vi "メイン.vi"() -> (2 "測定周期/ms":dbl, 3 "値転記用配列":T2[](array[typedef]))   [LabVIEW 2021] (continued)
                          n2295 = Add(x=w4469, y=13) -> (x+y=w4460:i32)
                          n2296 = local read "csv作成表"() -> (w4456:string[][])
                          n2297 = Unbundle By Name(w4467) -> ("実測値(MAX)"=w4463:string, "実測値(MIN)"=w4464:string)
                          n2298 = Replace Array Subset(array=w4456, new element #1=w4463, index (row) #1=w4461, index (col) #1=w4462, new element #2=w4464, index (row) #2=w4461, index (col) #2=w4460) -> (w4458:string[][])
                          n2299 = Select(t=w4458, s=w4468, f=w4456) -> (s? t:f=w4459:string[][])
                          n2300 = local write "csv作成表"(w4459) -> ()
                        }
                        frame 11 {
                          w4479 = 2
                          # "B"
                          # "A"
                          # "csv作成の為表へクラスタ(実測値)書き込み"
                          # "⑤"
                          # "③"
                          # "④"
                          n2301 = local read "メインON/OFF_\n設定 12"() -> (w4490:T1)
                          n2302 = Unbundle By Name(w4490) -> ("使用ON/OFF"=w4486:bool)
                          n2303 = control-ref of="前回値転記用配列"() -> (w4484:refnum<vi>)
                          n2304 = local read "メイン設定_設定 12"() -> (w4491:T2)
                          n2305 = call "メイン_測定値配列_CSV転記サブ.vi"("メイン設定_設定入力"=w4491, "ループ反復数値入力"=w4488, "実測設定項目"=w4489, "使用ON/OFF"=w4486, "前回値転記用配列"=w4484) -> ("ループ反復数値出力"=w4487:i32, "メイン設定_設定出力"=w4485:T2)  [unwired: 5 in]
                          n2306 = local write "メイン設定_設定 12"(w4485) -> ()
                          n2307 = Add(x=13, y=w4487) -> (x+y=w4480:i32)
                          n2308 = Add(x=w4487, y=14) -> (x+y=w4478:i32)
                          n2309 = local read "csv作成表"() -> (w4474:string[][])
                          n2310 = Unbundle By Name(w4485) -> ("実測値(MAX)"=w4481:string, "実測値(MIN)"=w4482:string)
                          n2311 = Replace Array Subset(array=w4474, new element #1=w4481, index (row) #1=w4479, index (col) #1=w4480, new element #2=w4482, index (row) #2=w4479, index (col) #2=w4478) -> (w4476:string[][])
                          n2312 = Select(t=w4476, s=w4486, f=w4474) -> (s? t:f=w4477:string[][])
                          n2313 = local write "csv作成表"(w4477) -> ()
                        }
                      }
                    }
                  }
                }
                n2314 = local write "値転記用配列"(w4248) -> ()
                n2315 = flat-sequence {
                  tunnel: [w4263] -> w4249
                  tunnel: w4248 -> [w4263]
                  frame #0 {
                    w4258 = T9 {"Horizontal"=-51, "Vertical"=216} ("座標 3")
                    n2316 = control-ref of="このVI"() -> (w4259:refnum<vi>)
                    n2317 = property on="ペーン 2" class="Pane"("Origin"=w4258) -> ()  [unwired: 2 in, 2 out]
                    n2318 = property on="ペーン 2" class="Pane"("Origin"=w4258) -> ()  [unwired: 2 in, 2 out]
                    n2319 = control-ref of="このVI"() -> (w4261:refnum<vi>)
                    n2320 = Unbundle(w4258) -> ("Vertical"=w4260:i16)  [unwired: 1 out]
                    n2321 = Unbundle(w4258) -> ("Vertical"=w4262:i16)  [unwired: 1 out]
                    n2322 = call "メイン_装飾移動サブ.vi"("Y軸座標入力"=w4260, "VI入力"=w4259) -> ()  [unwired: 10 in]
                    n2323 = call "メイン_装飾枠移動サブ.vi"("Y軸座標入力"=w4262, "VI入力"=w4261) -> ()  [unwired: 10 in]
                  }
                }
              }
              frame #1 {
                w4493 = T8."Enabled" ("無効")
                # "⑪ボタンの無効解除"
                n2324 = for {
                  N: 12 -> [_]
                  tunnel: w4493 -> [w4496]
                  i -> [w4497]
                  n2325 = case shown="11" w4497 {
                    tunnel: w4496 -> [w4498 w4499 w4500 w4501 w4502 w4503 w4504 w4505 w4506 w4507 w4508 w4509]
                    frame 0, Default {
                      n2326 = property on="メイン測定ボタン_単発 1" class="Bool (指定)"("DisabledEnum"=w4498) -> ()  [unwired: 2 in, 2 out]
                      n2327 = property on="メイン測定ボタン_連続 1" class="Bool (指定)"("DisabledEnum"=w4498) -> ()  [unwired: 2 in, 2 out]
                    }
                    frame 1 {
                      n2328 = property on="メイン測定ボタン_単発 2" class="Bool (指定)"("DisabledEnum"=w4499) -> ()  [unwired: 2 in, 2 out]
                      n2329 = property on="メイン測定ボタン_連続 2" class="Bool (指定)"("DisabledEnum"=w4499) -> ()  [unwired: 2 in, 2 out]
                    }
                    frame 2 {
                      n2330 = property on="メイン測定ボタン_単発 3" class="Bool (指定)"("DisabledEnum"=w4500) -> ()  [unwired: 2 in, 2 out]
                      n2331 = property on="メイン測定ボタン_連続 3" class="Bool (指定)"("DisabledEnum"=w4500) -> ()  [unwired: 2 in, 2 out]
                    }
                    frame 3 {
                      n2332 = property on="メイン測定ボタン_単発 4" class="Bool (指定)"("DisabledEnum"=w4501) -> ()  [unwired: 2 in, 2 out]
                      n2333 = property on="メイン測定ボタン_連続 4" class="Bool (指定)"("DisabledEnum"=w4501) -> ()  [unwired: 2 in, 2 out]
                    }
                    frame 4 {
                      n2334 = property on="メイン測定ボタン_単発 5" class="Bool (指定)"("DisabledEnum"=w4502) -> ()  [unwired: 2 in, 2 out]
                      n2335 = property on="メイン測定ボタン_連続 5" class="Bool (指定)"("DisabledEnum"=w4502) -> ()  [unwired: 2 in, 2 out]
                    }
                    frame 5 {
                      n2336 = property on="メイン測定ボタン_連続 6" class="Bool (指定)"("DisabledEnum"=w4503) -> ()  [unwired: 2 in, 2 out]
                      n2337 = property on="メイン測定ボタン_単発 6" class="Bool (指定)"("DisabledEnum"=w4503) -> ()  [unwired: 2 in, 2 out]
                    }
                    frame 6 {
                      n2338 = property on="メイン測定ボタン_連続 7" class="Bool (指定)"("DisabledEnum"=w4504) -> ()  [unwired: 2 in, 2 out]
                      n2339 = property on="メイン測定ボタン_単発 7" class="Bool (指定)"("DisabledEnum"=w4504) -> ()  [unwired: 2 in, 2 out]
                    }
                    frame 7 {
                      n2340 = property on="メイン測定ボタン_単発 8" class="Bool (指定)"("DisabledEnum"=w4505) -> ()  [unwired: 2 in, 2 out]
                      n2341 = property on="メイン測定ボタン_連続 8" class="Bool (指定)"("DisabledEnum"=w4505) -> ()  [unwired: 2 in, 2 out]
                    }
                    frame 8 {
                      n2342 = property on="メイン測定ボタン_単発 9" class="Bool (指定)"("DisabledEnum"=w4506) -> ()  [unwired: 2 in, 2 out]
                      n2343 = property on="メイン測定ボタン_連続 9" class="Bool (指定)"("DisabledEnum"=w4506) -> ()  [unwired: 2 in, 2 out]
                    }
                    frame 9 {
                      n2344 = property on="メイン測定ボタン_単発 10" class="Bool (指定)"("DisabledEnum"=w4507) -> ()  [unwired: 2 in, 2 out]
                      n2345 = property on="メイン測定ボタン_連続 10" class="Bool (指定)"("DisabledEnum"=w4507) -> ()  [unwired: 2 in, 2 out]
                    }
                    frame 10 {
                      n2346 = property on="メイン測定ボタン_単発 11" class="Bool (指定)"("DisabledEnum"=w4508) -> ()  [unwired: 2 in, 2 out]
                      n2347 = property on="メイン測定ボタン_連続 11" class="Bool (指定)"("DisabledEnum"=w4508) -> ()  [unwired: 2 in, 2 out]
                    }
                    frame 11 {
                      n2348 = property on="メイン測定ボタン_連続 12" class="Bool (指定)"("DisabledEnum"=w4509) -> ()  [unwired: 2 in, 2 out]
                      n2349 = property on="メイン測定ボタン_単発 12" class="Bool (指定)"("DisabledEnum"=w4509) -> ()  [unwired: 2 in, 2 out]
                    }
                  }
                }
                n2350 = local write "測定新値\nリセット用 4"(TRUE) -> ()
                n2351 = property on="TOPページへ" class="Bool"("DisabledEnum"=w4493) -> ()  [unwired: 2 in, 2 out]
                n2352 = property on="保存して終了" class="Bool"("DisabledEnum"=w4493) -> ()  [unwired: 2 in, 2 out]
                n2353 = property on="保存せずに" class="Bool"("DisabledEnum"=w4493) -> ()  [unwired: 2 in, 2 out]
              }
            }
          }
          frame True {
          }
        }
      }
      frame "測定5" {
        # "⑦"
        # "項目別のボタンで測定を行う為、項目分必要"
        n2354 = local read "測定旧値 5"() -> (w4513:bool)
        n2355 = case shown="FALSE" w4513 {
          tunnel: w4511 -> [w4516 w4779]
          tunnel: [w4515 w4779] -> w4512
          frame False {
            n2356 = flat-sequence {
              tunnel: w4516 -> [w4526]
              tunnel: [w4518] -> w4514
              tunnel: [w4764] -> w4515
              tunnel: w4514 -> [w4764]
              frame #0 {
                # "※複製コピー時変更する項目\n①②\nローカル変数\n\n入れ子のケースストラクチャ\"2\"を複製\n\n0～数だけ変更する\n③④⑤\nローカル変数\n\n※AB\n行番号の変更をする必要がある\n\n--------------------------------\nこの後イベントストラクチャ複製する\n--------------------------------\nイベントストラクチャ複製後\n\n⑦⑧\nローカル変数\n⑨\n装飾体の位置設定\n-51は固定\n前ケースの数値+72\n⑩\n測定新値リセット用\nのボタンが複製されているので、\nフロントパネルを整理する\n⑪\nプロパティノード\nボタンの無効解除クリア以外全てのボタン対象"
                # "実測完了の簡易疑似コード\n\n1)測定モードが単発・連続、多点かで転記する配列を変える\n2)値転記用配列へ転記\n\nここからゲージ分を繰り返す必要がある\n\n3)配列0を取り出す\n4)配列0のポートNoを取り出す\n5)メイン測定_設定配列(測定1の対象配列)のポートNoと比較\n6)同じだったら処理をする。違ったら何もしない\n7)同じだったら配列0のメインON/OFF_設定1の使用ON/OFFがTrueかFalseか\nFlaseだったら前回値転記用配列から前回の値をメイン設定_設定へ転記\nTrueだったらメイン設定_設定の測定モードから\n0単発、1連続、3多点\nの処理を行う\n8)測定値をメイン設定_設定へ転記したら、前回転記用配列へ転記する"
                # "⑨"
                # "⑧"
                # "②"
                # "グループNO(表示上はポートNo)が同じだったら値を転記する\n\n測定した配列のグループNOと値転記用配列の他の指標グループNOを比較する\n＝だったら、対象の配列のON/OFFボタンがTrueか確認し、\nTrueだったら、測定モードによって、値かMAX、MINの数値を転記する\n\nグループNOが同じでなければ、転記しない(何もしない)"
                # "まず値転記用配列に測定の値を転記"
                # "実測定画面vi動作"
                n2357 = local read "メイン設定_設定 5"() -> (w4521:T2)
                n2358 = local read "測定新値 5"() -> (→"測定新値\nリセット用 5":bool)
                n2359 = local read "測定周期/ms"() -> (w4519:dbl)
                n2360 = Unbundle By Name(w4521) -> ("測定モード"=w4522:u16)
                n2361 = call "実測定画面.vi"("実測設定項目配列_\nメインからの転記"=w4526, "測定周期/ms_制御器"=w4519) -> ("実測設定項目配列_\nゲージIOへ転記用"=w4524:T2[], "実測設定項目配列_\n多点測定メイン転記用"=w4523:T2[])  [unwired: 11 in, 1 out]
                n2362 = case shown="1" w4522 {
                  tunnel: w4524 -> [w4533 w4534 _]
                  tunnel: [w4533 w4534 w4535] -> w4517
                  tunnel: w4523 -> [_ _ w4535]
                  frame 0, Default {
                  }
                  frame 1 {
                  }
                  frame 2 {
                  }
                }
                n2363 = for {
                  N: 32 -> [_]
                  tunnel: w4517 -> [w4542]
                  i -> [w4537]
                  # "①"
                  # "※複製コピーはこのケースで行う"
                  # "32回分"
                  # "比較する固定GNO"
                  n2364 = local read "メイン設定_設定 5"() -> (w4536:T2)
                  n2365 = Index Array(array=w4542, index=w4537) -> (element=w4541:T2)
                  n2366 = Unbundle By Name(w4536) -> ("ポートNo."=w4540:dbl)
                  n2367 = Unbundle By Name(w4541) -> ("ポートNo."=w4539:dbl)
                  n2368 = Equal?(x=w4540, y=w4539) -> (x = y?=w4538:bool)
                  n2369 = case shown="TRUE" w4538 {
                    tunnel: w4541 -> [_ w4544]
                    tunnel: w4537 -> [_ w4543]
                    frame False {
                    }
                    frame True {
                      n2370 = case shown="0, デフォルト" w4543 {
                        tunnel: w4544 -> [w4560 w4578 w4596 w4614 w4632 w4650 w4668 w4686 w4704 w4722 w4740 w4758]
                        tunnel: w4543 -> [w4559 w4577 w4595 w4613 w4631 w4649 w4667 w4685 w4703 w4721 w4739 w4757]
                        frame 0, Default {
                          w4550 = 2
                          # "B"
                          # "A"
                          # "csv作成の為表へクラスタ(実測値)書き込み"
                          # "⑤"
                          # "③"
                          # "④"
                          n2371 = local read "メインON/OFF_\n設定 1"() -> (w4561:T1)
                          n2372 = Unbundle By Name(w4561) -> ("使用ON/OFF"=w4557:bool)
                          n2373 = control-ref of="前回値転記用配列"() -> (w4555:refnum<vi>)
                          n2374 = local read "メイン設定_設定 1"() -> (w4562:T2)
                          n2375 = call "メイン_測定値配列_CSV転記サブ.vi"("メイン設定_設定入力"=w4562, "ループ反復数値入力"=w4559, "実測設定項目"=w4560, "使用ON/OFF"=w4557, "前回値転記用配列"=w4555) -> ("ループ反復数値出力"=w4558:i32, "メイン設定_設定出力"=w4556:T2)  [unwired: 5 in]
                          n2376 = local write "メイン設定_設定 1"(w4556) -> ()
                          n2377 = Add(x=2, y=w4558) -> (x+y=w4551:i32)
                          n2378 = Add(x=w4558, y=3) -> (x+y=w4549:i32)
                          n2379 = local read "csv作成表"() -> (w4545:string[][])
                          n2380 = Unbundle By Name(w4556) -> ("実測値(MAX)"=w4552:string, "実測値(MIN)"=w4553:string)
                          n2381 = Replace Array Subset(array=w4545, new element #1=w4552, index (row) #1=w4550, index (col) #1=w4551, new element #2=w4553, index (row) #2=w4550, index (col) #2=w4549) -> (w4547:string[][])
                          n2382 = Select(t=w4547, s=w4557, f=w4545) -> (s? t:f=w4548:string[][])
                          n2383 = local write "csv作成表"(w4548) -> ()
                        }
                        frame 1 {
                          w4568 = 2
                          # "B"
                          # "A"
                          # "csv作成の為表へクラスタ(実測値)書き込み"
                          # "⑤"
                          # "③"
                          # "④"
                          n2384 = local read "メインON/OFF_\n設定 2"() -> (w4579:T1)
                          n2385 = Unbundle By Name(w4579) -> ("使用ON/OFF"=w4575:bool)
                          n2386 = control-ref of="前回値転記用配列"() -> (w4573:refnum<vi>)
                          n2387 = local read "メイン設定_設定 2"() -> (w4580:T2)
                          n2388 = call "メイン_測定値配列_CSV転記サブ.vi"("メイン設定_設定入力"=w4580, "ループ反復数値入力"=w4577, "実測設定項目"=w4578, "使用ON/OFF"=w4575, "前回値転記用配列"=w4573) -> ("ループ反復数値出力"=w4576:i32, "メイン設定_設定出力"=w4574:T2)  [unwired: 5 in]
                          n2389 = local write "メイン設定_設定 2"(w4574) -> ()
                          n2390 = Add(x=3, y=w4576) -> (x+y=w4569:i32)
                          n2391 = Add(x=w4576, y=4) -> (x+y=w4567:i32)
                          n2392 = local read "csv作成表"() -> (w4563:string[][])
                          n2393 = Unbundle By Name(w4574) -> ("実測値(MAX)"=w4570:string, "実測値(MIN)"=w4571:string)
                          n2394 = Replace Array Subset(array=w4563, new element #1=w4570, index (row) #1=w4568, index (col) #1=w4569, new element #2=w4571, index (row) #2=w4568, index (col) #2=w4567) -> (w4565:string[][])
                          n2395 = Select(t=w4565, s=w4575, f=w4563) -> (s? t:f=w4566:string[][])
                          n2396 = local write "csv作成表"(w4566) -> ()
                        }
                        frame 2 {
                          w4586 = 2
                          # "B"
                          # "A"
                          # "csv作成の為表へクラスタ(実測値)書き込み"
                          # "⑤"
                          # "③"
                          # "④"
                          n2397 = local read "メインON/OFF_\n設定 3"() -> (w4597:T1)
                          n2398 = Unbundle By Name(w4597) -> ("使用ON/OFF"=w4593:bool)
                          n2399 = control-ref of="前回値転記用配列"() -> (w4591:refnum<vi>)
                          n2400 = local read "メイン設定_設定 3"() -> (w4598:T2)
                          n2401 = call "メイン_測定値配列_CSV転記サブ.vi"("メイン設定_設定入力"=w4598, "ループ反復数値入力"=w4595, "実測設定項目"=w4596, "使用ON/OFF"=w4593, "前回値転記用配列"=w4591) -> ("ループ反復数値出力"=w4594:i32, "メイン設定_設定出力"=w4592:T2)  [unwired: 5 in]
                          n2402 = local write "メイン設定_設定 3"(w4592) -> ()
                          n2403 = Add(x=4, y=w4594) -> (x+y=w4587:i32)
                          n2404 = Add(x=w4594, y=5) -> (x+y=w4585:i32)
                          n2405 = local read "csv作成表"() -> (w4581:string[][])
                          n2406 = Unbundle By Name(w4592) -> ("実測値(MAX)"=w4588:string, "実測値(MIN)"=w4589:string)
                          n2407 = Replace Array Subset(array=w4581, new element #1=w4588, index (row) #1=w4586, index (col) #1=w4587, new element #2=w4589, index (row) #2=w4586, index (col) #2=w4585) -> (w4583:string[][])
                          n2408 = Select(t=w4583, s=w4593, f=w4581) -> (s? t:f=w4584:string[][])
                          n2409 = local write "csv作成表"(w4584) -> ()
                        }
                        frame 3 {
                          w4604 = 2
                          # "B"
                          # "A"
                          # "csv作成の為表へクラスタ(実測値)書き込み"
                          # "⑤"
                          # "③"
                          # "④"
                          n2410 = local read "メインON/OFF_\n設定 4"() -> (w4615:T1)
                          n2411 = Unbundle By Name(w4615) -> ("使用ON/OFF"=w4611:bool)
                          n2412 = control-ref of="前回値転記用配列"() -> (w4609:refnum<vi>)
                          n2413 = local read "メイン設定_設定 4"() -> (w4616:T2)
                          n2414 = call "メイン_測定値配列_CSV転記サブ.vi"("メイン設定_設定入力"=w4616, "ループ反復数値入力"=w4613, "実測設定項目"=w4614, "使用ON/OFF"=w4611, "前回値転記用配列"=w4609) -> ("ループ反復数値出力"=w4612:i32, "メイン設定_設定出力"=w4610:T2)  [unwired: 5 in]
                          n2415 = local write "メイン設定_設定 4"(w4610) -> ()
                          n2416 = Add(x=5, y=w4612) -> (x+y=w4605:i32)
                          n2417 = Add(x=w4612, y=6) -> (x+y=w4603:i32)
                          n2418 = local read "csv作成表"() -> (w4599:string[][])
                          n2419 = Unbundle By Name(w4610) -> ("実測値(MAX)"=w4606:string, "実測値(MIN)"=w4607:string)
                          n2420 = Replace Array Subset(array=w4599, new element #1=w4606, index (row) #1=w4604, index (col) #1=w4605, new element #2=w4607, index (row) #2=w4604, index (col) #2=w4603) -> (w4601:string[][])
                          n2421 = Select(t=w4601, s=w4611, f=w4599) -> (s? t:f=w4602:string[][])
                          n2422 = local write "csv作成表"(w4602) -> ()
                        }
                        frame 4 {
                          w4622 = 2
                          # "B"
                          # "A"
                          # "csv作成の為表へクラスタ(実測値)書き込み"
                          # "⑤"
                          # "③"
                          # "④"
                          n2423 = local read "メインON/OFF_\n設定 5"() -> (w4633:T1)
                          n2424 = Unbundle By Name(w4633) -> ("使用ON/OFF"=w4629:bool)
                          n2425 = control-ref of="前回値転記用配列"() -> (w4627:refnum<vi>)
                          n2426 = local read "メイン設定_設定 5"() -> (w4634:T2)
                          n2427 = call "メイン_測定値配列_CSV転記サブ.vi"("メイン設定_設定入力"=w4634, "ループ反復数値入力"=w4631, "実測設定項目"=w4632, "使用ON/OFF"=w4629, "前回値転記用配列"=w4627) -> ("ループ反復数値出力"=w4630:i32, "メイン設定_設定出力"=w4628:T2)  [unwired: 5 in]
                          n2428 = local write "メイン設定_設定 5"(w4628) -> ()
                          n2429 = Add(x=6, y=w4630) -> (x+y=w4623:i32)
                          n2430 = Add(x=w4630, y=7) -> (x+y=w4621:i32)
                          n2431 = local read "csv作成表"() -> (w4617:string[][])
                          n2432 = Unbundle By Name(w4628) -> ("実測値(MAX)"=w4624:string, "実測値(MIN)"=w4625:string)
                          n2433 = Replace Array Subset(array=w4617, new element #1=w4624, index (row) #1=w4622, index (col) #1=w4623, new element #2=w4625, index (row) #2=w4622, index (col) #2=w4621) -> (w4619:string[][])
                          n2434 = Select(t=w4619, s=w4629, f=w4617) -> (s? t:f=w4620:string[][])
                          n2435 = local write "csv作成表"(w4620) -> ()
                        }
                        frame 5 {
                          w4640 = 2
                          # "B"
                          # "A"
                          # "csv作成の為表へクラスタ(実測値)書き込み"
                          # "⑤"
                          # "③"
                          # "④"
                          n2436 = local read "メインON/OFF_\n設定 6"() -> (w4651:T1)
                          n2437 = Unbundle By Name(w4651) -> ("使用ON/OFF"=w4647:bool)
                          n2438 = control-ref of="前回値転記用配列"() -> (w4645:refnum<vi>)
                          n2439 = local read "メイン設定_設定 6"() -> (w4652:T2)
                          n2440 = call "メイン_測定値配列_CSV転記サブ.vi"("メイン設定_設定入力"=w4652, "ループ反復数値入力"=w4649, "実測設定項目"=w4650, "使用ON/OFF"=w4647, "前回値転記用配列"=w4645) -> ("ループ反復数値出力"=w4648:i32, "メイン設定_設定出力"=w4646:T2)  [unwired: 5 in]
                          n2441 = local write "メイン設定_設定 6"(w4646) -> ()
                          n2442 = Add(x=7, y=w4648) -> (x+y=w4641:i32)
                          n2443 = Add(x=w4648, y=8) -> (x+y=w4639:i32)
                          n2444 = local read "csv作成表"() -> (w4635:string[][])
                          n2445 = Unbundle By Name(w4646) -> ("実測値(MAX)"=w4642:string, "実測値(MIN)"=w4643:string)
                          n2446 = Replace Array Subset(array=w4635, new element #1=w4642, index (row) #1=w4640, index (col) #1=w4641, new element #2=w4643, index (row) #2=w4640, index (col) #2=w4639) -> (w4637:string[][])
                          n2447 = Select(t=w4637, s=w4647, f=w4635) -> (s? t:f=w4638:string[][])
                          n2448 = local write "csv作成表"(w4638) -> ()
                        }
                        frame 6 {
                          w4658 = 2
                          # "B"
                          # "A"
                          # "csv作成の為表へクラスタ(実測値)書き込み"
                          # "⑤"
                          # "③"
                          # "④"
                          n2449 = local read "メインON/OFF_\n設定 7"() -> (w4669:T1)
                          n2450 = Unbundle By Name(w4669) -> ("使用ON/OFF"=w4665:bool)
                          n2451 = control-ref of="前回値転記用配列"() -> (w4663:refnum<vi>)
                          n2452 = local read "メイン設定_設定 7"() -> (w4670:T2)
                          n2453 = call "メイン_測定値配列_CSV転記サブ.vi"("メイン設定_設定入力"=w4670, "ループ反復数値入力"=w4667, "実測設定項目"=w4668, "使用ON/OFF"=w4665, "前回値転記用配列"=w4663) -> ("ループ反復数値出力"=w4666:i32, "メイン設定_設定出力"=w4664:T2)  [unwired: 5 in]
                          n2454 = local write "メイン設定_設定 7"(w4664) -> ()
                          n2455 = Add(x=8, y=w4666) -> (x+y=w4659:i32)
                          n2456 = Add(x=w4666, y=9) -> (x+y=w4657:i32)
                          n2457 = local read "csv作成表"() -> (w4653:string[][])
                          n2458 = Unbundle By Name(w4664) -> ("実測値(MAX)"=w4660:string, "実測値(MIN)"=w4661:string)
                          n2459 = Replace Array Subset(array=w4653, new element #1=w4660, index (row) #1=w4658, index (col) #1=w4659, new element #2=w4661, index (row) #2=w4658, index (col) #2=w4657) -> (w4655:string[][])
                          n2460 = Select(t=w4655, s=w4665, f=w4653) -> (s? t:f=w4656:string[][])
                          n2461 = local write "csv作成表"(w4656) -> ()
                        }
                        frame 7 {
                          w4676 = 2
                          # "B"
                          # "A"
                          # "csv作成の為表へクラスタ(実測値)書き込み"
                          # "⑤"
                          # "③"
                          # "④"
                          n2462 = local read "メインON/OFF_\n設定 8"() -> (w4687:T1)
                          n2463 = Unbundle By Name(w4687) -> ("使用ON/OFF"=w4683:bool)
                          n2464 = control-ref of="前回値転記用配列"() -> (w4681:refnum<vi>)
                          n2465 = local read "メイン設定_設定 8"() -> (w4688:T2)
                          n2466 = call "メイン_測定値配列_CSV転記サブ.vi"("メイン設定_設定入力"=w4688, "ループ反復数値入力"=w4685, "実測設定項目"=w4686, "使用ON/OFF"=w4683, "前回値転記用配列"=w4681) -> ("ループ反復数値出力"=w4684:i32, "メイン設定_設定出力"=w4682:T2)  [unwired: 5 in]
                          n2467 = local write "メイン設定_設定 8"(w4682) -> ()
                          n2468 = Add(x=9, y=w4684) -> (x+y=w4677:i32)
                          n2469 = Add(x=w4684, y=10) -> (x+y=w4675:i32)
                          n2470 = local read "csv作成表"() -> (w4671:string[][])
                          n2471 = Unbundle By Name(w4682) -> ("実測値(MAX)"=w4678:string, "実測値(MIN)"=w4679:string)
                          n2472 = Replace Array Subset(array=w4671, new element #1=w4678, index (row) #1=w4676, index (col) #1=w4677, new element #2=w4679, index (row) #2=w4676, index (col) #2=w4675) -> (w4673:string[][])
                          n2473 = Select(t=w4673, s=w4683, f=w4671) -> (s? t:f=w4674:string[][])
                          n2474 = local write "csv作成表"(w4674) -> ()
                        }
                        frame 8 {
                          w4694 = 2
                          # "B"
                          # "A"
                          # "csv作成の為表へクラスタ(実測値)書き込み"
                          # "⑤"
                          # "③"
                          # "④"
                          n2475 = local read "メインON/OFF_\n設定 9"() -> (w4705:T1)
                          n2476 = Unbundle By Name(w4705) -> ("使用ON/OFF"=w4701:bool)
                          n2477 = control-ref of="前回値転記用配列"() -> (w4699:refnum<vi>)
                          n2478 = local read "メイン設定_設定 9"() -> (w4706:T2)
                          n2479 = call "メイン_測定値配列_CSV転記サブ.vi"("メイン設定_設定入力"=w4706, "ループ反復数値入力"=w4703, "実測設定項目"=w4704, "使用ON/OFF"=w4701, "前回値転記用配列"=w4699) -> ("ループ反復数値出力"=w4702:i32, "メイン設定_設定出力"=w4700:T2)  [unwired: 5 in]
                          n2480 = local write "メイン設定_設定 9"(w4700) -> ()
                          n2481 = Add(x=10, y=w4702) -> (x+y=w4695:i32)
                          n2482 = Add(x=w4702, y=11) -> (x+y=w4693:i32)
                          n2483 = local read "csv作成表"() -> (w4689:string[][])
                          n2484 = Unbundle By Name(w4700) -> ("実測値(MAX)"=w4696:string, "実測値(MIN)"=w4697:string)
                          n2485 = Replace Array Subset(array=w4689, new element #1=w4696, index (row) #1=w4694, index (col) #1=w4695, new element #2=w4697, index (row) #2=w4694, index (col) #2=w4693) -> (w4691:string[][])
                          n2486 = Select(t=w4691, s=w4701, f=w4689) -> (s? t:f=w4692:string[][])
                          n2487 = local write "csv作成表"(w4692) -> ()
                        }
                        frame 9 {
                          w4712 = 2
                          # "B"
                          # "A"
                          # "csv作成の為表へクラスタ(実測値)書き込み"
                          # "⑤"
                          # "③"
                          # "④"
                          n2488 = local read "メインON/OFF_\n設定 10"() -> (w4723:T1)
                          n2489 = Unbundle By Name(w4723) -> ("使用ON/OFF"=w4719:bool)
                          n2490 = control-ref of="前回値転記用配列"() -> (w4717:refnum<vi>)
                          n2491 = local read "メイン設定_設定 10"() -> (w4724:T2)
                          n2492 = call "メイン_測定値配列_CSV転記サブ.vi"("メイン設定_設定入力"=w4724, "ループ反復数値入力"=w4721, "実測設定項目"=w4722, "使用ON/OFF"=w4719, "前回値転記用配列"=w4717) -> ("ループ反復数値出力"=w4720:i32, "メイン設定_設定出力"=w4718:T2)  [unwired: 5 in]
                          n2493 = local write "メイン設定_設定 10"(w4718) -> ()
                          n2494 = Add(x=11, y=w4720) -> (x+y=w4713:i32)
                          n2495 = Add(x=w4720, y=12) -> (x+y=w4711:i32)
                          n2496 = local read "csv作成表"() -> (w4707:string[][])
                          n2497 = Unbundle By Name(w4718) -> ("実測値(MAX)"=w4714:string, "実測値(MIN)"=w4715:string)
                          n2498 = Replace Array Subset(array=w4707, new element #1=w4714, index (row) #1=w4712, index (col) #1=w4713, new element #2=w4715, index (row) #2=w4712, index (col) #2=w4711) -> (w4709:string[][])
                          n2499 = Select(t=w4709, s=w4719, f=w4707) -> (s? t:f=w4710:string[][])
                          n2500 = local write "csv作成表"(w4710) -> ()
                        }
                        frame 10 {
                          w4730 = 2
                          # "B"
                          # "A"
                          # "csv作成の為表へクラスタ(実測値)書き込み"
                          # "⑤"
                          # "③"
                          # "④"
                          n2501 = local read "メインON/OFF_\n設定 11"() -> (w4741:T1)
                          n2502 = Unbundle By Name(w4741) -> ("使用ON/OFF"=w4737:bool)
                          n2503 = control-ref of="前回値転記用配列"() -> (w4735:refnum<vi>)
                          n2504 = local read "メイン設定_設定 11"() -> (w4742:T2)
                          n2505 = call "メイン_測定値配列_CSV転記サブ.vi"("メイン設定_設定入力"=w4742, "ループ反復数値入力"=w4739, "実測設定項目"=w4740, "使用ON/OFF"=w4737, "前回値転記用配列"=w4735) -> ("ループ反復数値出力"=w4738:i32, "メイン設定_設定出力"=w4736:T2)  [unwired: 5 in]
                          n2506 = local write "メイン設定_設定 11"(w4736) -> ()
                          n2507 = Add(x=12, y=w4738) -> (x+y=w4731:i32)
                          n2508 = Add(x=w4738, y=13) -> (x+y=w4729:i32)
                          n2509 = local read "csv作成表"() -> (w4725:string[][])
                          n2510 = Unbundle By Name(w4736) -> ("実測値(MAX)"=w4732:string, "実測値(MIN)"=w4733:string)
                          n2511 = Replace Array Subset(array=w4725, new element #1=w4732, index (row) #1=w4730, index (col) #1=w4731, new element #2=w4733, index (row) #2=w4730, index (col) #2=w4729) -> (w4727:string[][])
                          n2512 = Select(t=w4727, s=w4737, f=w4725) -> (s? t:f=w4728:string[][])
                          n2513 = local write "csv作成表"(w4728) -> ()
                        }
                        frame 11 {
                          w4748 = 2
                          # "B"
                          # "A"
                          # "csv作成の為表へクラスタ(実測値)書き込み"
                          # "⑤"
                          # "③"
                          # "④"
                          n2514 = local read "メインON/OFF_\n設定 12"() -> (w4759:T1)
                          n2515 = Unbundle By Name(w4759) -> ("使用ON/OFF"=w4755:bool)
                          n2516 = control-ref of="前回値転記用配列"() -> (w4753:refnum<vi>)
                          n2517 = local read "メイン設定_設定 12"() -> (w4760:T2)
                          n2518 = call "メイン_測定値配列_CSV転記サブ.vi"("メイン設定_設定入力"=w4760, "ループ反復数値入力"=w4757, "実測設定項目"=w4758, "使用ON/OFF"=w4755, "前回値転記用配列"=w4753) -> ("ループ反復数値出力"=w4756:i32, "メイン設定_設定出力"=w4754:T2)  [unwired: 5 in]
                          n2519 = local write "メイン設定_設定 12"(w4754) -> ()
                          n2520 = Add(x=13, y=w4756) -> (x+y=w4749:i32)
                          n2521 = Add(x=w4756, y=14) -> (x+y=w4747:i32)
                          n2522 = local read "csv作成表"() -> (w4743:string[][])
                          n2523 = Unbundle By Name(w4754) -> ("実測値(MAX)"=w4750:string, "実測値(MIN)"=w4751:string)
                          n2524 = Replace Array Subset(array=w4743, new element #1=w4750, index (row) #1=w4748, index (col) #1=w4749, new element #2=w4751, index (row) #2=w4748, index (col) #2=w4747) -> (w4745:string[][])
                          n2525 = Select(t=w4745, s=w4755, f=w4743) -> (s? t:f=w4746:string[][])
                          n2526 = local write "csv作成表"(w4746) -> ()
                        }
                      }
                    }
                  }
                }
                n2527 = local write "値転記用配列"(w4517) -> ()
                n2528 = flat-sequence {
                  tunnel: [w4532] -> w4518
                  tunnel: w4517 -> [w4532]
                  frame #0 {
                    w4527 = T9 {"Horizontal"=-51, "Vertical"=288} ("座標 4")
                    n2529 = control-ref of="このVI"() -> (w4528:refnum<vi>)
                    n2530 = property on="ペーン 2" class="Pane"("Origin"=w4527) -> ()  [unwired: 2 in, 2 out]
                    n2531 = property on="ペーン 2" class="Pane"("Origin"=w4527) -> ()  [unwired: 2 in, 2 out]
                    n2532 = control-ref of="このVI"() -> (w4530:refnum<vi>)
                    n2533 = Unbundle(w4527) -> ("Vertical"=w4529:i16)  [unwired: 1 out]
                    n2534 = Unbundle(w4527) -> ("Vertical"=w4531:i16)  [unwired: 1 out]
                    n2535 = call "メイン_装飾移動サブ.vi"("Y軸座標入力"=w4529, "VI入力"=w4528) -> ()  [unwired: 10 in]
                    n2536 = call "メイン_装飾枠移動サブ.vi"("Y軸座標入力"=w4531, "VI入力"=w4530) -> ()  [unwired: 10 in]
                  }
                }
              }
              frame #1 {
                w4762 = T8."Enabled" ("無効")
                # "⑪ボタンの無効解除"
                n2537 = for {
                  N: 12 -> [_]
                  tunnel: w4762 -> [w4765]
                  i -> [w4766]
                  n2538 = case shown="11" w4766 {
                    tunnel: w4765 -> [w4767 w4768 w4769 w4770 w4771 w4772 w4773 w4774 w4775 w4776 w4777 w4778]
                    frame 0, Default {
                      n2539 = property on="メイン測定ボタン_単発 1" class="Bool (指定)"("DisabledEnum"=w4767) -> ()  [unwired: 2 in, 2 out]
                      n2540 = property on="メイン測定ボタン_連続 1" class="Bool (指定)"("DisabledEnum"=w4767) -> ()  [unwired: 2 in, 2 out]
                    }
                    frame 1 {
                      n2541 = property on="メイン測定ボタン_単発 2" class="Bool (指定)"("DisabledEnum"=w4768) -> ()  [unwired: 2 in, 2 out]
                      n2542 = property on="メイン測定ボタン_連続 2" class="Bool (指定)"("DisabledEnum"=w4768) -> ()  [unwired: 2 in, 2 out]
                    }
                    frame 2 {
                      n2543 = property on="メイン測定ボタン_単発 3" class="Bool (指定)"("DisabledEnum"=w4769) -> ()  [unwired: 2 in, 2 out]
                      n2544 = property on="メイン測定ボタン_連続 3" class="Bool (指定)"("DisabledEnum"=w4769) -> ()  [unwired: 2 in, 2 out]
                    }
                    frame 3 {
                      n2545 = property on="メイン測定ボタン_単発 4" class="Bool (指定)"("DisabledEnum"=w4770) -> ()  [unwired: 2 in, 2 out]
                      n2546 = property on="メイン測定ボタン_連続 4" class="Bool (指定)"("DisabledEnum"=w4770) -> ()  [unwired: 2 in, 2 out]
                    }
                    frame 4 {
                      n2547 = property on="メイン測定ボタン_単発 5" class="Bool (指定)"("DisabledEnum"=w4771) -> ()  [unwired: 2 in, 2 out]
                      n2548 = property on="メイン測定ボタン_連続 5" class="Bool (指定)"("DisabledEnum"=w4771) -> ()  [unwired: 2 in, 2 out]
                    }
                    frame 5 {
                      n2549 = property on="メイン測定ボタン_連続 6" class="Bool (指定)"("DisabledEnum"=w4772) -> ()  [unwired: 2 in, 2 out]
                      n2550 = property on="メイン測定ボタン_単発 6" class="Bool (指定)"("DisabledEnum"=w4772) -> ()  [unwired: 2 in, 2 out]
                    }
                    frame 6 {
                      n2551 = property on="メイン測定ボタン_連続 7" class="Bool (指定)"("DisabledEnum"=w4773) -> ()  [unwired: 2 in, 2 out]
                      n2552 = property on="メイン測定ボタン_単発 7" class="Bool (指定)"("DisabledEnum"=w4773) -> ()  [unwired: 2 in, 2 out]
                    }
                    frame 7 {
                      n2553 = property on="メイン測定ボタン_単発 8" class="Bool (指定)"("DisabledEnum"=w4774) -> ()  [unwired: 2 in, 2 out]
                      n2554 = property on="メイン測定ボタン_連続 8" class="Bool (指定)"("DisabledEnum"=w4774) -> ()  [unwired: 2 in, 2 out]
                    }
                    frame 8 {
                      n2555 = property on="メイン測定ボタン_単発 9" class="Bool (指定)"("DisabledEnum"=w4775) -> ()  [unwired: 2 in, 2 out]
                      n2556 = property on="メイン測定ボタン_連続 9" class="Bool (指定)"("DisabledEnum"=w4775) -> ()  [unwired: 2 in, 2 out]
                    }
                    frame 9 {
                      n2557 = property on="メイン測定ボタン_単発 10" class="Bool (指定)"("DisabledEnum"=w4776) -> ()  [unwired: 2 in, 2 out]
                      n2558 = property on="メイン測定ボタン_連続 10" class="Bool (指定)"("DisabledEnum"=w4776) -> ()  [unwired: 2 in, 2 out]
                    }
                    frame 10 {
                      n2559 = property on="メイン測定ボタン_単発 11" class="Bool (指定)"("DisabledEnum"=w4777) -> ()  [unwired: 2 in, 2 out]
                      n2560 = property on="メイン測定ボタン_連続 11" class="Bool (指定)"("DisabledEnum"=w4777) -> ()  [unwired: 2 in, 2 out]
                    }
                    frame 11 {
                      n2561 = property on="メイン測定ボタン_連続 12" class="Bool (指定)"("DisabledEnum"=w4778) -> ()  [unwired: 2 in, 2 out]
                      n2562 = property on="メイン測定ボタン_単発 12" class="Bool (指定)"("DisabledEnum"=w4778) -> ()  [unwired: 2 in, 2 out]
                    }
                  }
                }
                n2563 = property on="TOPページへ" class="Bool"("DisabledEnum"=w4762) -> ()  [unwired: 2 in, 2 out]
                n2564 = property on="保存して終了" class="Bool"("DisabledEnum"=w4762) -> ()  [unwired: 2 in, 2 out]
                n2565 = property on="保存せずに" class="Bool"("DisabledEnum"=w4762) -> ()  [unwired: 2 in, 2 out]
                n2566 = local write "測定新値\nリセット用 5"(TRUE) -> ()
              }
            }
          }
          frame True {
          }
        }
      }
      frame "測定6" {
        # "⑦"
        # "項目別のボタンで測定を行う為、項目分必要"
        n2567 = local read "測定旧値 6"() -> (w4782:bool)
        n2568 = case shown="FALSE" w4782 {
          tunnel: w4780 -> [w4785 w5048]
          tunnel: [w4784 w5048] -> w4781
          frame False {
            n2569 = flat-sequence {
              tunnel: w4785 -> [w4795]
              tunnel: [w4787] -> w4783
              tunnel: [w5033] -> w4784
              tunnel: w4783 -> [w5033]
              frame #0 {
                # "※複製コピー時変更する項目\n①②\nローカル変数\n\n入れ子のケースストラクチャ\"2\"を複製\n\n0～数だけ変更する\n③④⑤\nローカル変数\n\n※AB\n行番号の変更をする必要がある\n\n--------------------------------\nこの後イベントストラクチャ複製する\n--------------------------------\nイベントストラクチャ複製後\n\n⑦⑧\nローカル変数\n⑨\n装飾体の位置設定\n-51は固定\n前ケースの数値+72\n⑩\n測定新値リセット用\nのボタンが複製されているので、\nフロントパネルを整理する\n⑪\nプロパティノード\nボタンの無効解除クリア以外全てのボタン対象"
                # "実測完了の簡易疑似コード\n\n1)測定モードが単発・連続、多点かで転記する配列を変える\n2)値転記用配列へ転記\n\nここからゲージ分を繰り返す必要がある\n\n3)配列0を取り出す\n4)配列0のポートNoを取り出す\n5)メイン測定_設定配列(測定1の対象配列)のポートNoと比較\n6)同じだったら処理をする。違ったら何もしない\n7)同じだったら配列0のメインON/OFF_設定1の使用ON/OFFがTrueかFalseか\nFlaseだったら前回値転記用配列から前回の値をメイン設定_設定へ転記\nTrueだったらメイン設定_設定の測定モードから\n0単発、1連続、3多点\nの処理を行う\n8)測定値をメイン設定_設定へ転記したら、前回転記用配列へ転記する"
                # "⑨"
                # "⑧"
                # "②"
                # "グループNO(表示上はポートNo)が同じだったら値を転記する\n\n測定した配列のグループNOと値転記用配列の他の指標グループNOを比較する\n＝だったら、対象の配列のON/OFFボタンがTrueか確認し、\nTrueだったら、測定モードによって、値かMAX、MINの数値を転記する\n\nグループNOが同じでなければ、転記しない(何もしない)"
                # "まず値転記用配列に測定の値を転記"
                # "実測定画面vi動作"
                n2570 = local read "メイン設定_設定 6"() -> (w4790:T2)
                n2571 = local read "測定新値 6"() -> (→"測定新値\nリセット用 6":bool)
                n2572 = local read "測定周期/ms"() -> (w4788:dbl)
                n2573 = Unbundle By Name(w4790) -> ("測定モード"=w4791:u16)
                n2574 = call "実測定画面.vi"("実測設定項目配列_\nメインからの転記"=w4795, "測定周期/ms_制御器"=w4788) -> ("実測設定項目配列_\nゲージIOへ転記用"=w4793:T2[], "実測設定項目配列_\n多点測定メイン転記用"=w4792:T2[])  [unwired: 11 in, 1 out]
                n2575 = case shown="1" w4791 {
                  tunnel: w4793 -> [w4802 w4803 _]
                  tunnel: [w4802 w4803 w4804] -> w4786
                  tunnel: w4792 -> [_ _ w4804]
                  frame 0, Default {
                  }
                  frame 1 {
                  }
                  frame 2 {
                  }
                }
                n2576 = for {
                  N: 32 -> [_]
                  tunnel: w4786 -> [w4811]
                  i -> [w4806]
                  # "①"
                  # "※複製コピーはこのケースで行う"
                  # "32回分"
                  # "比較する固定GNO"
                  n2577 = local read "メイン設定_設定 6"() -> (w4805:T2)
                  n2578 = Index Array(array=w4811, index=w4806) -> (element=w4810:T2)
                  n2579 = Unbundle By Name(w4805) -> ("ポートNo."=w4809:dbl)
                  n2580 = Unbundle By Name(w4810) -> ("ポートNo."=w4808:dbl)
                  n2581 = Equal?(x=w4809, y=w4808) -> (x = y?=w4807:bool)
                  n2582 = case shown="TRUE" w4807 {
                    tunnel: w4810 -> [_ w4813]
                    tunnel: w4806 -> [_ w4812]
                    frame False {
                    }
                    frame True {
                      n2583 = case shown="0, デフォルト" w4812 {
                        tunnel: w4813 -> [w4829 w4847 w4865 w4883 w4901 w4919 w4937 w4955 w4973 w4991 w5009 w5027]
                        tunnel: w4812 -> [w4828 w4846 w4864 w4882 w4900 w4918 w4936 w4954 w4972 w4990 w5008 w5026]
                        frame 0, Default {
                          w4819 = 2
                          # "B"
                          # "A"
                          # "csv作成の為表へクラスタ(実測値)書き込み"
                          # "⑤"
                          # "③"
                          # "④"
                          n2584 = local read "メインON/OFF_\n設定 1"() -> (w4830:T1)
                          n2585 = Unbundle By Name(w4830) -> ("使用ON/OFF"=w4826:bool)
                          n2586 = control-ref of="前回値転記用配列"() -> (w4824:refnum<vi>)
                          n2587 = local read "メイン設定_設定 1"() -> (w4831:T2)
                          n2588 = call "メイン_測定値配列_CSV転記サブ.vi"("メイン設定_設定入力"=w4831, "ループ反復数値入力"=w4828, "実測設定項目"=w4829, "使用ON/OFF"=w4826, "前回値転記用配列"=w4824) -> ("ループ反復数値出力"=w4827:i32, "メイン設定_設定出力"=w4825:T2)  [unwired: 5 in]
                          n2589 = local write "メイン設定_設定 1"(w4825) -> ()
                          n2590 = Add(x=2, y=w4827) -> (x+y=w4820:i32)
                          n2591 = Add(x=w4827, y=3) -> (x+y=w4818:i32)
                          n2592 = local read "csv作成表"() -> (w4814:string[][])
                          n2593 = Unbundle By Name(w4825) -> ("実測値(MAX)"=w4821:string, "実測値(MIN)"=w4822:string)
                          n2594 = Replace Array Subset(array=w4814, new element #1=w4821, index (row) #1=w4819, index (col) #1=w4820, new element #2=w4822, index (row) #2=w4819, index (col) #2=w4818) -> (w4816:string[][])
                          n2595 = Select(t=w4816, s=w4826, f=w4814) -> (s? t:f=w4817:string[][])
                          n2596 = local write "csv作成表"(w4817) -> ()
                        }
                        frame 1 {
                          w4837 = 2
                          # "B"
                          # "A"
                          # "csv作成の為表へクラスタ(実測値)書き込み"
                          # "⑤"
                          # "③"
                          # "④"
                          n2597 = local read "メインON/OFF_\n設定 2"() -> (w4848:T1)
                          n2598 = Unbundle By Name(w4848) -> ("使用ON/OFF"=w4844:bool)
                          n2599 = control-ref of="前回値転記用配列"() -> (w4842:refnum<vi>)
                          n2600 = local read "メイン設定_設定 2"() -> (w4849:T2)
                          n2601 = call "メイン_測定値配列_CSV転記サブ.vi"("メイン設定_設定入力"=w4849, "ループ反復数値入力"=w4846, "実測設定項目"=w4847, "使用ON/OFF"=w4844, "前回値転記用配列"=w4842) -> ("ループ反復数値出力"=w4845:i32, "メイン設定_設定出力"=w4843:T2)  [unwired: 5 in]
                          n2602 = local write "メイン設定_設定 2"(w4843) -> ()
                          n2603 = Add(x=3, y=w4845) -> (x+y=w4838:i32)
                          n2604 = Add(x=w4845, y=4) -> (x+y=w4836:i32)
                          n2605 = local read "csv作成表"() -> (w4832:string[][])
                          n2606 = Unbundle By Name(w4843) -> ("実測値(MAX)"=w4839:string, "実測値(MIN)"=w4840:string)
                          n2607 = Replace Array Subset(array=w4832, new element #1=w4839, index (row) #1=w4837, index (col) #1=w4838, new element #2=w4840, index (row) #2=w4837, index (col) #2=w4836) -> (w4834:string[][])
                          n2608 = Select(t=w4834, s=w4844, f=w4832) -> (s? t:f=w4835:string[][])
                          n2609 = local write "csv作成表"(w4835) -> ()
                        }
                        frame 2 {
                          w4855 = 2
                          # "B"
                          # "A"
                          # "csv作成の為表へクラスタ(実測値)書き込み"
                          # "⑤"
                          # "③"
                          # "④"
                          n2610 = local read "メインON/OFF_\n設定 3"() -> (w4866:T1)
                          n2611 = Unbundle By Name(w4866) -> ("使用ON/OFF"=w4862:bool)
                          n2612 = control-ref of="前回値転記用配列"() -> (w4860:refnum<vi>)
                          n2613 = local read "メイン設定_設定 3"() -> (w4867:T2)
                          n2614 = call "メイン_測定値配列_CSV転記サブ.vi"("メイン設定_設定入力"=w4867, "ループ反復数値入力"=w4864, "実測設定項目"=w4865, "使用ON/OFF"=w4862, "前回値転記用配列"=w4860) -> ("ループ反復数値出力"=w4863:i32, "メイン設定_設定出力"=w4861:T2)  [unwired: 5 in]
                          n2615 = local write "メイン設定_設定 3"(w4861) -> ()
                          n2616 = Add(x=4, y=w4863) -> (x+y=w4856:i32)
                          n2617 = Add(x=w4863, y=5) -> (x+y=w4854:i32)
                          n2618 = local read "csv作成表"() -> (w4850:string[][])
                          n2619 = Unbundle By Name(w4861) -> ("実測値(MAX)"=w4857:string, "実測値(MIN)"=w4858:string)
                          n2620 = Replace Array Subset(array=w4850, new element #1=w4857, index (row) #1=w4855, index (col) #1=w4856, new element #2=w4858, index (row) #2=w4855, index (col) #2=w4854) -> (w4852:string[][])
                          n2621 = Select(t=w4852, s=w4862, f=w4850) -> (s? t:f=w4853:string[][])
                          n2622 = local write "csv作成表"(w4853) -> ()
                        }
                        frame 3 {
                          w4873 = 2
                          # "B"
                          # "A"
                          # "csv作成の為表へクラスタ(実測値)書き込み"
                          # "⑤"
                          # "③"
                          # "④"
                          n2623 = local read "メインON/OFF_\n設定 4"() -> (w4884:T1)
                          n2624 = Unbundle By Name(w4884) -> ("使用ON/OFF"=w4880:bool)
                          n2625 = control-ref of="前回値転記用配列"() -> (w4878:refnum<vi>)
                          n2626 = local read "メイン設定_設定 4"() -> (w4885:T2)
                          n2627 = call "メイン_測定値配列_CSV転記サブ.vi"("メイン設定_設定入力"=w4885, "ループ反復数値入力"=w4882, "実測設定項目"=w4883, "使用ON/OFF"=w4880, "前回値転記用配列"=w4878) -> ("ループ反復数値出力"=w4881:i32, "メイン設定_設定出力"=w4879:T2)  [unwired: 5 in]
                          n2628 = local write "メイン設定_設定 4"(w4879) -> ()
                          n2629 = Add(x=5, y=w4881) -> (x+y=w4874:i32)
                          n2630 = Add(x=w4881, y=6) -> (x+y=w4872:i32)
                          n2631 = local read "csv作成表"() -> (w4868:string[][])
                          n2632 = Unbundle By Name(w4879) -> ("実測値(MAX)"=w4875:string, "実測値(MIN)"=w4876:string)
                          n2633 = Replace Array Subset(array=w4868, new element #1=w4875, index (row) #1=w4873, index (col) #1=w4874, new element #2=w4876, index (row) #2=w4873, index (col) #2=w4872) -> (w4870:string[][])
                          n2634 = Select(t=w4870, s=w4880, f=w4868) -> (s? t:f=w4871:string[][])
                          n2635 = local write "csv作成表"(w4871) -> ()
                        }
                        frame 4 {
                          w4891 = 2
                          # "B"
                          # "A"
                          # "csv作成の為表へクラスタ(実測値)書き込み"
                          # "⑤"
                          # "③"
                          # "④"
                          n2636 = local read "メインON/OFF_\n設定 5"() -> (w4902:T1)
                          n2637 = Unbundle By Name(w4902) -> ("使用ON/OFF"=w4898:bool)
                          n2638 = control-ref of="前回値転記用配列"() -> (w4896:refnum<vi>)
                          n2639 = local read "メイン設定_設定 5"() -> (w4903:T2)
                          n2640 = call "メイン_測定値配列_CSV転記サブ.vi"("メイン設定_設定入力"=w4903, "ループ反復数値入力"=w4900, "実測設定項目"=w4901, "使用ON/OFF"=w4898, "前回値転記用配列"=w4896) -> ("ループ反復数値出力"=w4899:i32, "メイン設定_設定出力"=w4897:T2)  [unwired: 5 in]
                          n2641 = local write "メイン設定_設定 5"(w4897) -> ()
                          n2642 = Add(x=6, y=w4899) -> (x+y=w4892:i32)
                          n2643 = Add(x=w4899, y=7) -> (x+y=w4890:i32)
                          n2644 = local read "csv作成表"() -> (w4886:string[][])
                          n2645 = Unbundle By Name(w4897) -> ("実測値(MAX)"=w4893:string, "実測値(MIN)"=w4894:string)
                          n2646 = Replace Array Subset(array=w4886, new element #1=w4893, index (row) #1=w4891, index (col) #1=w4892, new element #2=w4894, index (row) #2=w4891, index (col) #2=w4890) -> (w4888:string[][])
                          n2647 = Select(t=w4888, s=w4898, f=w4886) -> (s? t:f=w4889:string[][])
                          n2648 = local write "csv作成表"(w4889) -> ()
                        }
                        frame 5 {
                          w4909 = 2
                          # "B"
                          # "A"
                          # "csv作成の為表へクラスタ(実測値)書き込み"
                          # "⑤"
                          # "③"
                          # "④"
                          n2649 = local read "メインON/OFF_\n設定 6"() -> (w4920:T1)
                          n2650 = Unbundle By Name(w4920) -> ("使用ON/OFF"=w4916:bool)
                          n2651 = control-ref of="前回値転記用配列"() -> (w4914:refnum<vi>)
                          n2652 = local read "メイン設定_設定 6"() -> (w4921:T2)
                          n2653 = call "メイン_測定値配列_CSV転記サブ.vi"("メイン設定_設定入力"=w4921, "ループ反復数値入力"=w4918, "実測設定項目"=w4919, "使用ON/OFF"=w4916, "前回値転記用配列"=w4914) -> ("ループ反復数値出力"=w4917:i32, "メイン設定_設定出力"=w4915:T2)  [unwired: 5 in]
                          n2654 = local write "メイン設定_設定 6"(w4915) -> ()
                          n2655 = Add(x=7, y=w4917) -> (x+y=w4910:i32)
                          n2656 = Add(x=w4917, y=8) -> (x+y=w4908:i32)
                          n2657 = local read "csv作成表"() -> (w4904:string[][])
                          n2658 = Unbundle By Name(w4915) -> ("実測値(MAX)"=w4911:string, "実測値(MIN)"=w4912:string)
                          n2659 = Replace Array Subset(array=w4904, new element #1=w4911, index (row) #1=w4909, index (col) #1=w4910, new element #2=w4912, index (row) #2=w4909, index (col) #2=w4908) -> (w4906:string[][])
                          n2660 = Select(t=w4906, s=w4916, f=w4904) -> (s? t:f=w4907:string[][])
                          n2661 = local write "csv作成表"(w4907) -> ()
                        }
                        frame 6 {
                          w4927 = 2
                          # "B"
                          # "A"
                          # "csv作成の為表へクラスタ(実測値)書き込み"
                          # "⑤"
                          # "③"
                          # "④"
                          n2662 = local read "メインON/OFF_\n設定 7"() -> (w4938:T1)
                          n2663 = Unbundle By Name(w4938) -> ("使用ON/OFF"=w4934:bool)
                          n2664 = control-ref of="前回値転記用配列"() -> (w4932:refnum<vi>)
                          n2665 = local read "メイン設定_設定 7"() -> (w4939:T2)
                          n2666 = call "メイン_測定値配列_CSV転記サブ.vi"("メイン設定_設定入力"=w4939, "ループ反復数値入力"=w4936, "実測設定項目"=w4937, "使用ON/OFF"=w4934, "前回値転記用配列"=w4932) -> ("ループ反復数値出力"=w4935:i32, "メイン設定_設定出力"=w4933:T2)  [unwired: 5 in]
                          n2667 = local write "メイン設定_設定 7"(w4933) -> ()
                          n2668 = Add(x=8, y=w4935) -> (x+y=w4928:i32)
                          n2669 = Add(x=w4935, y=9) -> (x+y=w4926:i32)
                          n2670 = local read "csv作成表"() -> (w4922:string[][])
                          n2671 = Unbundle By Name(w4933) -> ("実測値(MAX)"=w4929:string, "実測値(MIN)"=w4930:string)
                          n2672 = Replace Array Subset(array=w4922, new element #1=w4929, index (row) #1=w4927, index (col) #1=w4928, new element #2=w4930, index (row) #2=w4927, index (col) #2=w4926) -> (w4924:string[][])
                          n2673 = Select(t=w4924, s=w4934, f=w4922) -> (s? t:f=w4925:string[][])
                          n2674 = local write "csv作成表"(w4925) -> ()
                        }
                        frame 7 {
                          w4945 = 2
                          # "B"
                          # "A"
                          # "csv作成の為表へクラスタ(実測値)書き込み"
                          # "⑤"
                          # "③"
                          # "④"
                          n2675 = local read "メインON/OFF_\n設定 8"() -> (w4956:T1)
                          n2676 = Unbundle By Name(w4956) -> ("使用ON/OFF"=w4952:bool)
                          n2677 = control-ref of="前回値転記用配列"() -> (w4950:refnum<vi>)
                          n2678 = local read "メイン設定_設定 8"() -> (w4957:T2)
                          n2679 = call "メイン_測定値配列_CSV転記サブ.vi"("メイン設定_設定入力"=w4957, "ループ反復数値入力"=w4954, "実測設定項目"=w4955, "使用ON/OFF"=w4952, "前回値転記用配列"=w4950) -> ("ループ反復数値出力"=w4953:i32, "メイン設定_設定出力"=w4951:T2)  [unwired: 5 in]
                          n2680 = local write "メイン設定_設定 8"(w4951) -> ()
                          n2681 = Add(x=9, y=w4953) -> (x+y=w4946:i32)
                          n2682 = Add(x=w4953, y=10) -> (x+y=w4944:i32)
                          n2683 = local read "csv作成表"() -> (w4940:string[][])
                          n2684 = Unbundle By Name(w4951) -> ("実測値(MAX)"=w4947:string, "実測値(MIN)"=w4948:string)
                          n2685 = Replace Array Subset(array=w4940, new element #1=w4947, index (row) #1=w4945, index (col) #1=w4946, new element #2=w4948, index (row) #2=w4945, index (col) #2=w4944) -> (w4942:string[][])
                          n2686 = Select(t=w4942, s=w4952, f=w4940) -> (s? t:f=w4943:string[][])
                          n2687 = local write "csv作成表"(w4943) -> ()
                        }
                        frame 8 {
                          w4963 = 2
                          # "B"
                          # "A"
                          # "csv作成の為表へクラスタ(実測値)書き込み"
                          # "⑤"
                          # "③"
                          # "④"
                          n2688 = local read "メインON/OFF_\n設定 9"() -> (w4974:T1)
                          n2689 = Unbundle By Name(w4974) -> ("使用ON/OFF"=w4970:bool)
                          n2690 = control-ref of="前回値転記用配列"() -> (w4968:refnum<vi>)
                          n2691 = local read "メイン設定_設定 9"() -> (w4975:T2)
                          n2692 = call "メイン_測定値配列_CSV転記サブ.vi"("メイン設定_設定入力"=w4975, "ループ反復数値入力"=w4972, "実測設定項目"=w4973, "使用ON/OFF"=w4970, "前回値転記用配列"=w4968) -> ("ループ反復数値出力"=w4971:i32, "メイン設定_設定出力"=w4969:T2)  [unwired: 5 in]
                          n2693 = local write "メイン設定_設定 9"(w4969) -> ()
                          n2694 = Add(x=10, y=w4971) -> (x+y=w4964:i32)
                          n2695 = Add(x=w4971, y=11) -> (x+y=w4962:i32)
                          n2696 = local read "csv作成表"() -> (w4958:string[][])
                          n2697 = Unbundle By Name(w4969) -> ("実測値(MAX)"=w4965:string, "実測値(MIN)"=w4966:string)
                          n2698 = Replace Array Subset(array=w4958, new element #1=w4965, index (row) #1=w4963, index (col) #1=w4964, new element #2=w4966, index (row) #2=w4963, index (col) #2=w4962) -> (w4960:string[][])
                          n2699 = Select(t=w4960, s=w4970, f=w4958) -> (s? t:f=w4961:string[][])
                          n2700 = local write "csv作成表"(w4961) -> ()
                        }
                        frame 9 {
                          w4981 = 2
                          # "B"
                          # "A"
